vi "Remove Invalid Characters.vi"(10 "String":string, 11 "Character Position Possible Letters":T1) -> (3 "Updated Character Position":string[](array[string]))   [LabVIEW 2025, in "WordleSolver.lvlib"]
uses:
  WordleSolver.lvlib
  Controls/Character Position Possible Letters.ctl
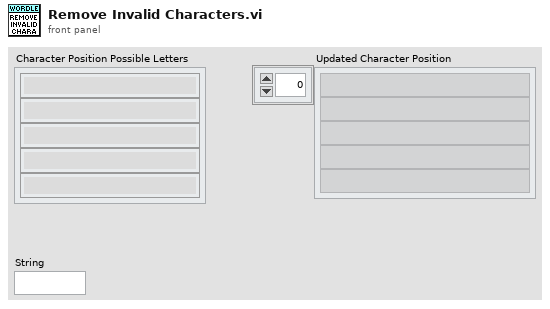
[diagram p1: front panel]
types:
  T1 = typedef "Character Position Possible Letters.ctl" = string[]
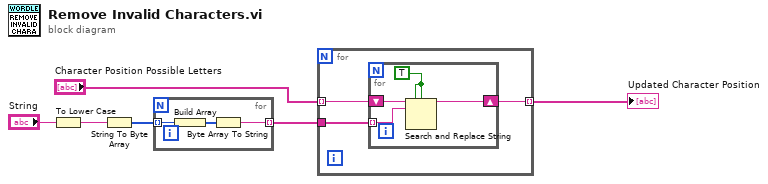
[diagram p0: block diagram]
diagram:
  n1 = To Lower Case(string="String") -> (all lower case string=w1:string)
  n2 = String To Byte Array(string=w1) -> (unsigned byte array=w4:u8[])
  n3 = for {
    tunnel: w4 -> [w9] mode=indexing
    tunnel: [w7] -> w5 mode=indexing
    n4 = Build Array(w9) -> (w8:u8[])
    n5 = Byte Array To String(unsigned byte array=w8) -> (string=w7:string)
  }
  n6 = for {
    tunnel: "Character Position Possible Letters" -> [w12] mode=indexing
    tunnel: w5 -> [w11]
    tunnel: [w10] -> w6 mode=indexing
    n7 = for {
      tunnel: w11 -> [w15] mode=indexing
      shift-right: [w13] -> w10
      shift-left: w12 -> [w16]
      w14 = TRUE ("ignore case? (F)")
      n8 = Search and Replace String(replace all?=w14, case sensitive?=w14, input string=w16, search string=w15) -> (result string=w13:string)  [unwired: 4 in, 3 out]
    }
  }
  "Updated Character Position" <- w6
